vi "Build Two Term Compare Types.vi"(11 "Comparison Name":string) -> ()   [LabVIEW 2019]
uses:
  <vilib>/numeric/LVNumericRepresentation.ctl
  71b9e51f-dfc8-458f-9837-ddab78837e89.vi
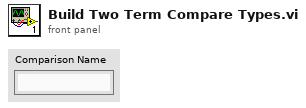
[diagram p1: front panel]
types:
  T1 = typedef "LVNumericRepresentation.ctl" = enum32{"Extended Precision", "Double Precision", "Single Precision", "Long", "Word", "Byte", "Unsigned Long", "Unsigned Word", "Unsigned Byte", "Complex Extended", "Complex Double", "Complex Single", "Quad", "Unsigned Quad", "Fixed-Point"}
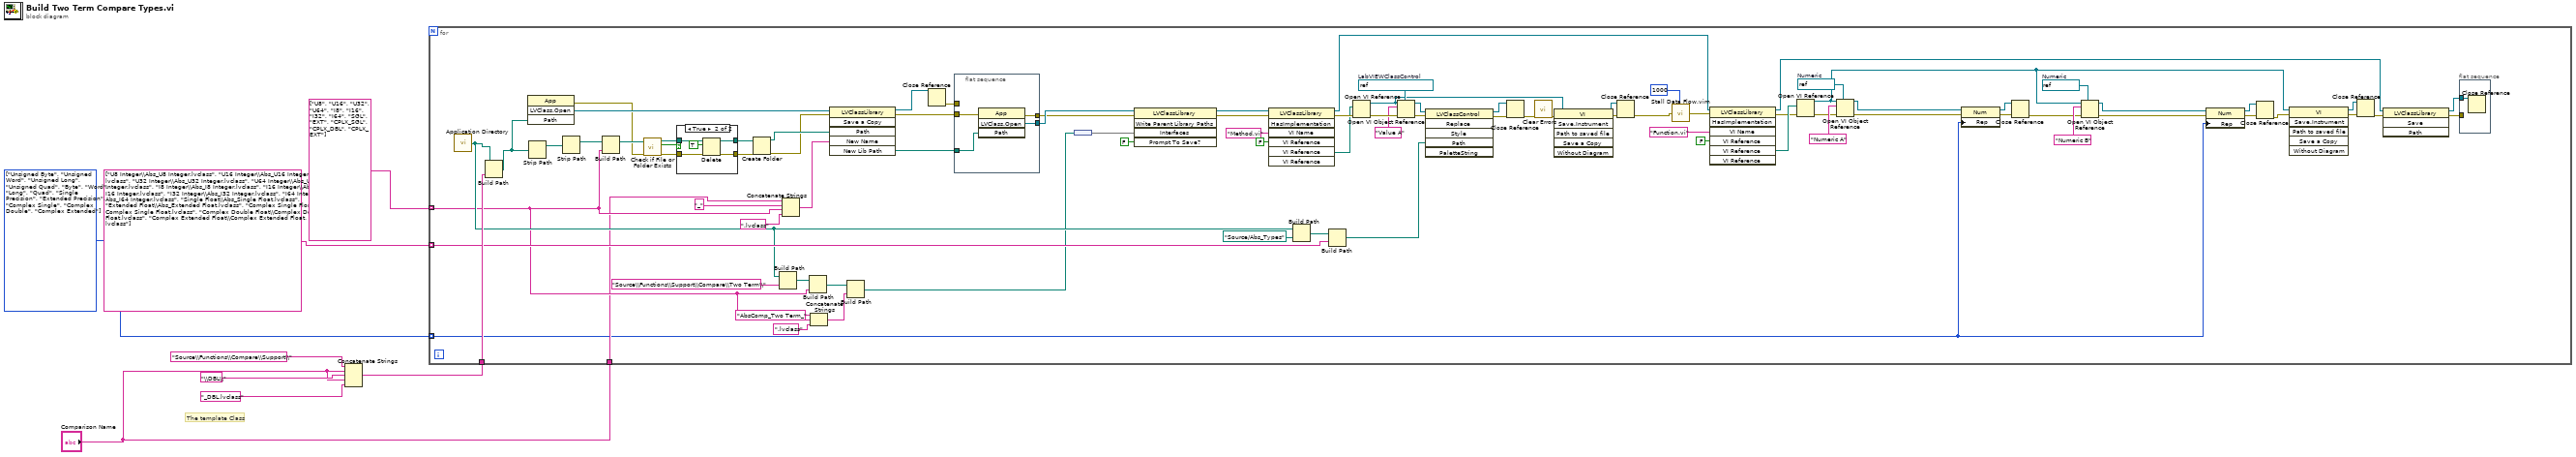
[diagram p0: block diagram]
diagram:
  w6 = T1[] [enum."Unsigned Byte", enum."Unsigned Word", enum."Unsigned Long", enum."Unsigned Quad", enum."Byte", enum."Word", enum."Long", enum."Quad", enum."Single Precision", enum."Extended Precision", enum."Complex Single", enum."Complex Double", enum."Complex Extended"] items=["Extended Precision", "Double Precision", "Single Precision", "Long", "Word", "Byte", "Unsigned Long", "Unsigned Word", "Unsigned Byte", "Complex Extended", "Complex Double", "Complex Single", "Quad", "Unsigned Quad", "Fixed-Point"] ("Representation")
  # "The template Class"
  n1 = Concatenate Strings("Source\\Functions\\Compare\\Support\\", "Comparison Name", "\\DBL\\", "Comparison Name", "_DBL.lvclass") -> (w2:string)
  n2 = for {
    tunnel: string[] ["U8", "U16", "U32", "U64", "I8", "I16", "I32", "I64", "SGL", "EXT", "CPLX_SGL", "CPLX_DBL", "CPLX_EXT"] -> [w33] mode=indexing
    tunnel: w2 -> [w77]
    tunnel: string[] ["U8 Integer\\Abs_U8 Integer.lvclass", "U16 Integer\\Abs_U16 Integer.lvclass", "U32 Integer\\Abs_U32 Integer.lvclass", "U64 Integer\\Abs_U64 Integer.lvclass", "I8 Integer\\Abs_I8 Integer.lvclass", "I16 Integer\\Abs_I16 Integer.lvclass", "I32 Integer\\Abs_I32 Integer.lvclass", "I64 Integer\\Abs_I64 Integer.lvclass", "Single Float\\Abs_Single Float.lvclass", "Extended Float\\Abs_Extended Float.lvclass", "Complex Single Float\\Complex Single Float.lvclass", "Complex Double Float\\Complex Double Float.lvclass", "Complex Extended Float\\Complex Extended Float.lvclass"] -> [w69] mode=indexing
    tunnel: w6 -> [w10] mode=indexing
    tunnel: "Comparison Name" -> [w19]
    w14 = refnum<vi> refnum  # Numeric
    w54 = refnum<vi> refnum  # Numeric
    w63 = refnum<vi> refnum  # LabVIEWClassControl
    n3 = call <vilib>:"Application Directory.vi"() -> ("Application Directory"=w37:path)
    n4 = Build Path(base path=w37, name or relative path=w77) -> (appended path=w78:path)
    n5 = invoke class="App" method="LVClass.Open"("Path"=w78) -> (error out=w83:errorcluster, "LVClass.Open"=w96:refnum<vi>)  [unwired: 3 in, 2 out]
    n6 = Strip Path(path=w78) -> (stripped path=w94:path)  [unwired: 1 out]
    n7 = Strip Path(path=w94) -> (stripped path=w93:path)  [unwired: 1 out]
    n8 = Build Path(base path=w93, name or relative path=w33) -> (appended path=w89:path)
    n9 = call <vilib>:"Check if File or Folder Exists.vi"("error in (no error)"=w83, "path"=w89) -> ("error out"=w82:errorcluster, "file or folder exists?"=w91:bool, "dup path"=w92:path)  [unwired: 7 in]
    n10 = case shown="True" w91 {
      tunnel: w92 -> [w103 w108]
      tunnel: [w103 w106] -> w90
      tunnel: w82 -> [w102 w105]
      tunnel: [w102 w104] -> w81
      frame False {
      }
      frame True {
        n11 = Delete(path (use dialog)=w108, entire hierarchy (F)=TRUE, error in=w105) -> (deleted path=w106:path, error out=w104:errorcluster)  [unwired: 2 in, 1 out]
      }
    }
    n12 = Create Folder(path (use dialog)=w90, error in=w81) -> (created path=w88:path, error out=w80:errorcluster)  [unwired: 1 in, 1 out]
    n13 = Build Path(base path=w37, name or relative path="Source\\Functions\\Support\\Compare\\Two Term\\") -> (appended path=w36:path)
    n14 = Concatenate Strings(w19, "_", w33, ".lvclass") -> (w76:string)
    n15 = Build Path(base path=w36, name or relative path=w33) -> (appended path=w35:path)
    n16 = Concatenate Strings("AbsComp_Two Term_" ("string"), w33, ".lvclass") -> (w31:string)
    n17 = invoke class="LVClassLibrary" method="Save a Copy"(reference=w96, error in=w80, "Path"=w88, "New Name"=w76) -> (reference out=w95:refnum<vi>, error out=w84:errorcluster, "New Lib Path"=w85:path)  [unwired: 2 in, 3 out]
    n18 = Build Path(base path=w35, name or relative path=w31) -> (appended path=w29:path)
    n19 = Close Reference(reference=w95) -> (error out=w79:errorcluster)  [unwired: 1 in]
    n20 = flat-sequence {
      tunnel: w85 -> [w100]
      tunnel: w84 -> [w101]
      tunnel: w79 -> [_]
      tunnel: [w98] -> w46
      tunnel: [w99] -> w30
      frame #0 {
        n21 = invoke class="App" method="LVClass.Open"(error in=w101, "Path"=w100) -> (error out=w99:errorcluster, "LVClass.Open"=w98:refnum<vi>)  [unwired: 2 in, 2 out]
      }
    }
    n22 = node(w29) -> (w28:set{path})
    n23 = invoke class="LVClassLibrary" method="Write Parent Library Paths"(reference=w46, error in=w30, "Interfaces"=w28, "Prompt To Save?"=FALSE) -> (reference out=w45:refnum<vi>, error out=w44:errorcluster)  [unwired: 1 in, 3 out]
    n24 = invoke class="LVClassLibrary" method="HasImplementation"(reference=w45, error in=w44, "VI Name"="Method.vi", "VI Reference"=FALSE ("Consider Parents?")) -> (reference out=w48:refnum<vi>, error out=w74:errorcluster, "VI Reference"=w73:path)  [unwired: 3 in, 4 out]
    n25 = Build Path(base path=w37, name or relative path=path "Source/Abs_Types") -> (appended path=w70:path)
    n26 = Build Path(base path=w70, name or relative path=w69) -> (appended path=w47:path)
    n27 = Open VI Reference(vi path=w73, error in (no error)=w74) -> (vi reference=w23:refnum<vi>, error out=w68:errorcluster)  [unwired: 4 in]
    n28 = Open VI Object Reference(7:w63, 8:w68, 10:"Value A" ("name/order"), 11:w23) -> (0:w66:errorcluster, 3:w65:refnum<vi>)
    n29 = invoke class="LVClassControl" method="Replace"(reference=w65, error in=w66, "Path"=w47) -> (reference out=w64:refnum<vi>, error out=w62:errorcluster)  [unwired: 3 in, 4 out]
    n30 = Close Reference(reference=w64, error in (no error)=w62) -> (error out=w61:errorcluster)
    n31 = call <vilib>:"Clear Errors.vi"("error in (no error)"=w61) -> ("error out"=w24:errorcluster)  [unwired: 5 in, 1 out]
    n32 = invoke class="VI" method="Save.Instrument"(reference=w23, error in=w24) -> (reference out=w22:refnum<vi>, error out=w25:errorcluster)  [unwired: 4 in, 4 out]
    n33 = Close Reference(reference=w22, error in (no error)=w25) -> (error out=w51:errorcluster)
    n34 = call "Stall Data Flow.vim"("value in"=w51, "milliseconds to wait"=u32 1000) -> ("value out"=w50:errorcluster)  [unwired: 1 out]
    n35 = invoke class="LVClassLibrary" method="HasImplementation"(reference=w48, error in=w50, "VI Name"="Function.vi", "VI Reference"=FALSE ("Consider Parents?")) -> (reference out=w40:refnum<vi>, error out=w57:errorcluster, "VI Reference"=w58:path)  [unwired: 3 in, 4 out]
    n36 = Open VI Reference(vi path=w58, error in (no error)=w57) -> (vi reference=w12:refnum<vi>, error out=w55:errorcluster)  [unwired: 4 in]
    n37 = Open VI Object Reference(7:w54, 8:w55, 10:"Numeric A" ("name/order"), 11:w12) -> (0:w26:errorcluster, 3:w27:refnum<vi>)
    n38 = property class="Num"(reference=w27, error in=w26, "Rep"=w10) -> (reference out=w52:refnum<vi>, error out=w53:errorcluster)
    n39 = Close Reference(reference=w52, error in (no error)=w53) -> (error out=w11:errorcluster)
    n40 = Open VI Object Reference(7:w14, 8:w11, 10:"Numeric B" ("name/order"), 11:w12) -> (0:w18:errorcluster, 3:w17:refnum<vi>)
    n41 = property class="Num"(reference=w17, error in=w18, "Rep"=w10) -> (reference out=w16:refnum<vi>, error out=w15:errorcluster)
    n42 = Close Reference(reference=w16, error in (no error)=w15) -> (error out=w9:errorcluster)
    n43 = invoke class="VI" method="Save.Instrument"(reference=w12, error in=w9) -> (reference out=w21:refnum<vi>, error out=w20:errorcluster)  [unwired: 4 in, 4 out]
    n44 = Close Reference(reference=w21, error in (no error)=w20) -> (error out=w42:errorcluster)
    n45 = invoke class="LVClassLibrary" method="Save"(reference=w40, error in=w42) -> (reference out=w39:refnum<vi>, error out=w41:errorcluster)  [unwired: 2 in, 2 out]
    n46 = flat-sequence {
      tunnel: w39 -> [w97]
      tunnel: w41 -> [_]
      frame #0 {
        n47 = Close Reference(reference=w97) -> ()  [unwired: 1 in, 1 out]
      }
    }
  }
